vi "Write Pref (STR).vi"(8 "error in (no error)":errorcluster, 9 "Value":string, 10 "Pref Hierarchy":string[](array[string]), 11 "Pref Group in":refnum<class "Pref Group.lvclass">) -> (0 "error out":errorcluster, 3 "Pref Group out":refnum<class "Pref Group.lvclass">)   [LabVIEW 2020, in "User Prefs.lvlib" / "Pref Group.lvclass"]
uses:
  Pref Group.lvclass
  PrefsDB/Write Pref Data.ctl
  lv-cdm/CDM-Config/Config Manager/Config Manager.lvclass
  lv-promises/Promises/Promise/Promise.lvclass
  lv-promises/Promises/No Parameter/No Parameter.lvclass
  C:/dev/lv20CE/relink/lv-promises/Promises/Value/Value.lvclass
  Pref Group.lvclass/Pref Group.ctl
  lv-promises/Promises/Promise/Promise.lvclass/Promise.ctl
  lv-promises/Promises/Future/Future.lvclass/Future.ctl
  lv-promises/Promises/Future/Future.lvclass
  User Prefs.lvlib
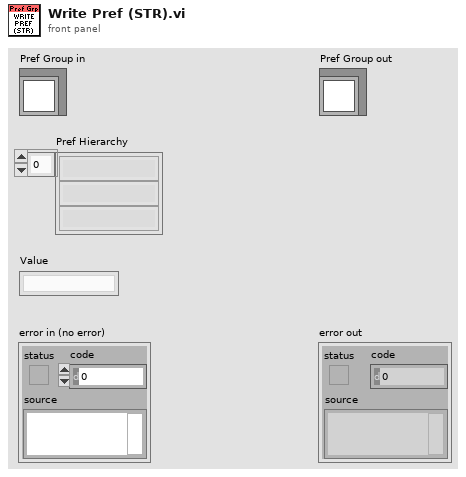
[diagram p1: front panel]
types:
  T1 = typedef "User Prefs.lvlib/Write Pref Data.ctl" = cluster{"Hierarchy":string[], "Value":string, "Config":refnum<class "Config Manager.lvclass">, "Promise":refnum<class "Promise.lvclass">}
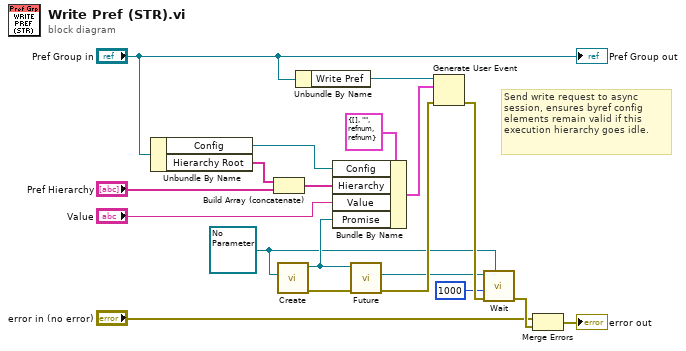
[diagram p0: block diagram]
diagram:
  w4 = refnum<class "No Parameter.lvclass"> refnum ("Futures:No Parameter.lvclass")
  # "Send write request to async session, ensures byref config elements remain valid if this execution hierarchy goes idle."
  n1 = Unbundle By Name("Pref Group in") -> ("Config"=w13:refnum<class "Config Manager.lvclass">, "Hierarchy Root"=w16:string[])
  n2 = Build Array (concatenate)(w16, "Pref Hierarchy") -> (w14:string[])
  n3 = call "Create.vi"("Result Type"=w4) -> ("error out"=w7:errorcluster, "Promise"=w11:refnum<class "Promise.lvclass">)  [unwired: 9 in]
  n4 = Unbundle By Name("Pref Group in") -> ("Write Pref"=w9:refnum<user-event>)
  n5 = Bundle By Name(cluster=T1 {"Hierarchy"=[], "Value"="", "Config"=refnum, "Promise"=refnum} ("Write Pref Data"), "Config"=w13, "Hierarchy"=w14, "Value"="Value", "Promise"=w11) -> (w8:T1)
  n6 = call "Future.vi"("Promise in"=w11) -> ("Future"=w6:refnum<class "Future.lvclass">)  [unwired: 9 in, 1 out]
  n7 = Generate User Event(user event=w9, event data cluster=w8, error in=w7) -> (error out=w18:errorcluster)  [unwired: 1 in, 1 out]
  n8 = call "Wait.vi"("Result Type"=w4, "error in (no error)"=w18, "Timeout mS (-1)"=1000, "Future in"=w6) -> ("error out"=w3:errorcluster)  [unwired: 6 in, 1 out]
  n9 = Merge Errors("error in (no error)", w3) -> (→"error out":errorcluster)
  "Pref Group out" <- "Pref Group in"
